vi "Continuous CCC.vi"() -> ()   [LabVIEW 2018]
uses:
  <vilib>/Rock Robotics/SystemInterfaces/i2clib/i2c_bus.ctl
  source/library/Interface/Pixy Com.lvclass
  source/deviceSupport/FRC/I2C/RoboRIO I2C.lvclass
  source/library/Pixy2.lvlib
  <vilib>/Rock Robotics/SystemInterfaces/spilib/spi_bus.ctl
  source/deviceSupport/FRC/SPI/RoboRIO SPI.lvclass
  source/deviceSupport/FRC/UART/RoboRIO UART.lvclass
  <vilib>/Rock Robotics/WPI/SerialPort/WPI_SerialPort.ctl
panel:
  in  "milliseconds to wait":u32
  in  "signature map":u8=255 format="%.0x"
  in  "max blocks":u8=255
  out "view":picture
  in  "Stop Button":bool
  out "error out":errorcluster
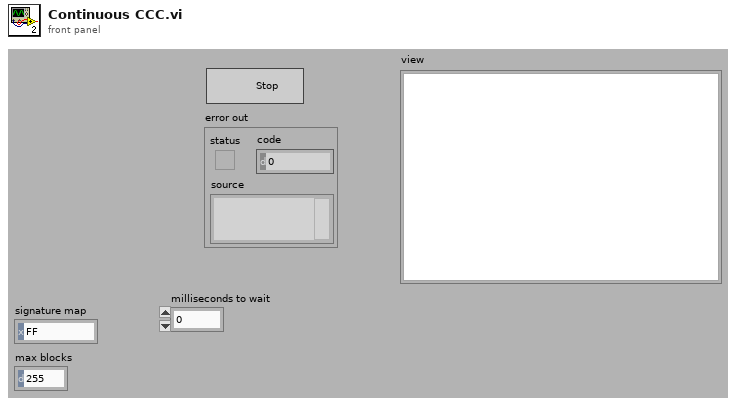
[diagram p1: front panel]
types:
  T1 = typedef "i2c_bus.ctl" = enum16{"I2C On-Board", "I2C MXP", "Invalid"}
  T2 = typedef "spi_bus.ctl" = enum16{"SPI On-Board, CS0", "SPI On-Board, CS1", "SPI On-Board, CS2", "SPI On-Board, CS3", "SPI MXP", "Invalid"}
  T3 = typedef "WPI_SerialPort.ctl" = enum16{"Onboard RS-232", "MXP TTL", "USB 1", "USB 2"}
  T4 = typedef "Pixy2.lvlib/Block.ctl" = cluster{"signature":u16, "x":u16, "y":u16, "width":u16, "height":u16, "angle":i16, "index":u8, "age":u8}
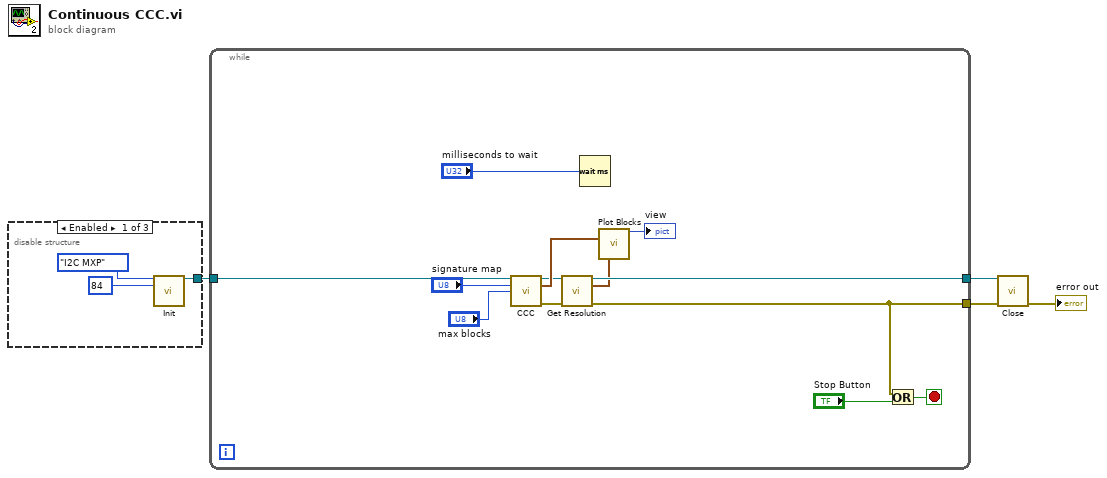
[diagram p0: block diagram]
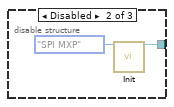
[diagram p2: hidden frame]
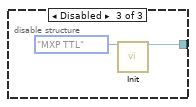
[diagram p3: hidden frame]
diagram:
  n1 = disable-structure shown="Enabled" {
    disable-tunnel: [w7 w9 w11] -> w4
    frame Enabled {
      n2 = call "Init.vi"("I2C bus"=i2c_bus."I2C MXP" ("I2C Bus"), "device address"=u8 84 ("Device Address")) -> ("comm interface out"=w7:refnum<class "Pixy Com.lvclass">)  [unwired: 12 in, 1 out]
    }
    frame Disabled {
      n3 = call "Init.vi"("SPI Bus"=spi_bus."SPI MXP") -> ("comm interface out"=w9:refnum<class "Pixy Com.lvclass">)  [unwired: 13 in, 1 out]
    }
    frame Disabled {
      n4 = call "Init.vi"("serial port"=WPI_SerialPort."MXP TTL") -> ("comm interface out"=w11:refnum<class "Pixy Com.lvclass">)  [unwired: 13 in, 1 out]
    }
  }
  n5 = while {
    tunnel: w4 -> [w24]
    tunnel: [w22] -> w3
    tunnel: [w23] -> w2
    stop <- w21 stop-if-true
    n6 = call "CCC.vi"("comm interface in"=w24, "signature map"="signature map", "max blocks"="max blocks") -> ("comm interface out"=w15:refnum<class "Pixy Com.lvclass">, "blocks"=w17:T4[], "error out"=w14:errorcluster)  [unwired: 10 in]
    n7 = call "Get Resolution.vi"("comm interface in"=w15, "error in"=w14) -> ("comm interface out"=w23:refnum<class "Pixy Com.lvclass">, "resolution"=w13:cluster{"width":u16, "height":u16}, "error out"=w22:errorcluster)  [unwired: 11 in]
    n8 = Wait (ms)(milliseconds to wait="milliseconds to wait") -> ()  [unwired: 1 out]
    n9 = call "Plot Blocks.vi"("blocks"=w17, "pixy resolution"=w13) -> ("picture out"=→"view":picture)  [unwired: 13 in]
    n10 = Or(x=w22, y="Stop Button") -> (x .or. y?=w21:bool)
  }
  n11 = call-dynamic "Close.vi"("comm interface in"=w2, "error in"=w3) -> ("error out"=→"error out":errorcluster)  [unwired: 13 in]
